vi "Read POS DEGREE.vi"(8 "error in (no error)":errorcluster, 11 "ParameterConf in":refnum<class "ParameterConf.lvclass">) -> (0 "error out":errorcluster, 1 "DEGREES":cluster{"X":dbl, "Y":dbl}, 2 "POS":cluster{"X":dbl, "Y":dbl, "Z":dbl}, 3 "ParameterConf out":refnum<class "ParameterConf.lvclass">)   [LabVIEW 2017, in "LibraryGcode.lvlib" / "ParameterConf.lvclass"]
uses:
  ParameterConf.lvclass
  ParameterConf.lvclass/ParameterConf.ctl
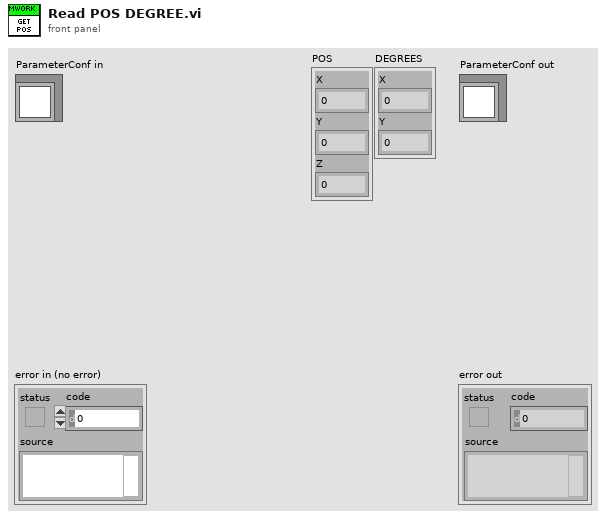
[diagram p1: front panel]
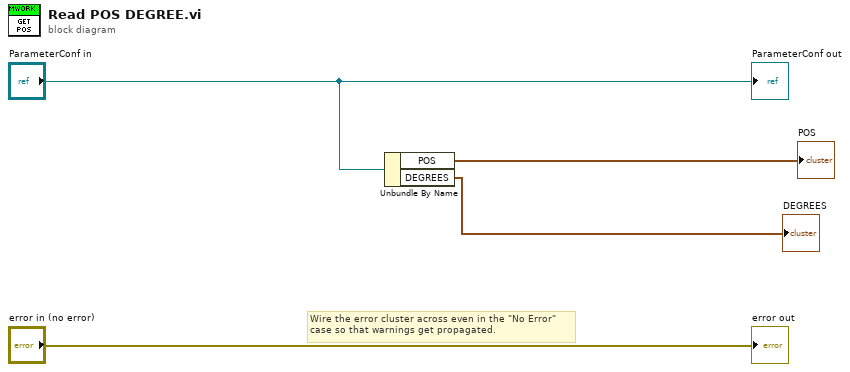
[diagram p0: block diagram]
diagram:
  # "Wire the error cluster across even in the \"No Error\"\ncase so that warnings get propagated."
  n1 = Unbundle By Name("ParameterConf in") -> ("POS"=→"POS":cluster{"X":dbl, "Y":dbl, "Z":dbl}, "DEGREES"=→"DEGREES":cluster{"X":dbl, "Y":dbl})
  "error out" <- "error in (no error)"
  "ParameterConf out" <- "ParameterConf in"
